vi "IMAQ Create.vi"(1 "Border Size":i32=3, 2 "Image Name":string="untitled", 5 "Image Type":T1 items=["Grayscale (U8)", "Grayscale (I16)", "Grayscale (SGL)", "Complex (CSG)", "RGB (U32)", "HSL (U32)", "RGB (U64)", "Grayscale (U16)"], 6 "error in (no error)":errorcluster) -> (0 "New Image":T2, 3 "error out":errorcluster)   [LabVIEW 2019]
doc: "Creates a temporary memory location for an image."
uses:
  <vilib>/vision/Image Controls.llb/IMAQ Image.ctl
  nivissvc.dll
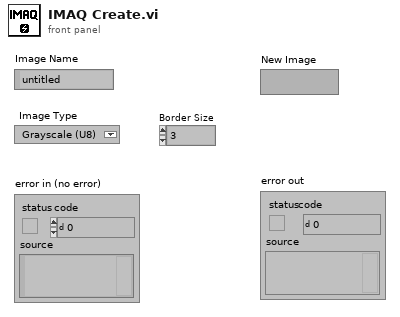
[diagram p1: front panel]
types:
  T1 = typedef "Image Type" = u32
  T2 = typedef "IMAQ Image.ctl" = refnum<image>
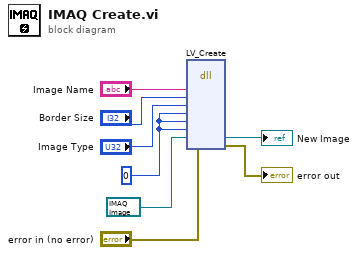
[diagram p0: block diagram]
diagram:
  w3 = 0
  n1 = dll-call lib="nivissvc.*" fn="LV_Create"("name"="Image Name", "border"="Border Size", "imageType"="Image Type", "width"=w3, "height"=w3, "lock space"=w3, "image"=T2 refnum ("New Image"), "err"="error in (no error)") -> ("image"=→"New Image":T2, "err"=→"error out":errorcluster)  [unwired: 9 in, 3 out]
